vi "IV_Reader_SweepScroller.vi"() -> ()   [LabVIEW 2016]
panel:
  in  "Sweep parameters":T1={"Vbg"=15.0, "Vbg step"=0.0, "Vsg"=-0.5, "Vsg step"=0.025, "B"=0.0, "B step"=0.0, "Temp"=2.0, "Temp step"=0.0}
  in  "PNG output folder":path=path "C:/Users/ansom/Desktop/Agilent/PNG's From Graphs/B_BG_7to-7"
  in  "Large Sweep Folder":path=path "B:/SketchSET/SA03008H.20180718/77_B+SG_B_-7to0inc1_SG_-0.5to0.5inc0.25_at0.2Hz_-300mVto-100mV_IV_@BG15"
  in  "# Fast Sweep":dbl=41.0
  in  "# Slow Sweep":dbl=8.0
  # "Vbg will be updated autmatically"
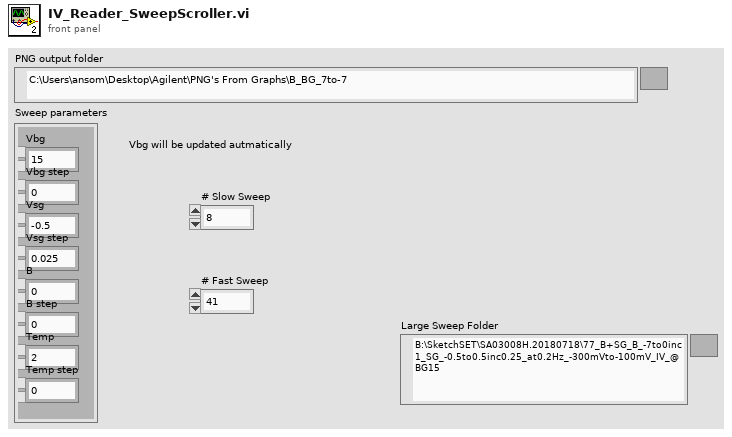
[diagram p1: front panel]
types:
  T1 = cluster{"Vbg":dbl, "Vbg step":dbl, "Vsg":dbl, "Vsg step":dbl, "B":dbl, "B step":dbl, "Temp":dbl, "Temp step":dbl}
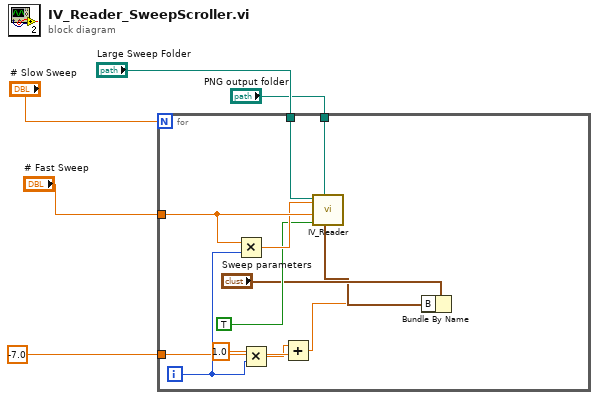
[diagram p0: block diagram]
diagram:
  n1 = for {
    N: "# Slow Sweep" -> [_]
    tunnel: "# Fast Sweep" -> [w17]
    tunnel: "Large Sweep Folder" -> [w15]
    tunnel: "PNG output folder" -> [w13]
    tunnel: -7.0 -> [w8]
    i -> [w9]
    n2 = Multiply(x=w17, y=w9) -> (x*y=w16:dbl)
    n3 = Multiply(x=1.0, y=w9) -> (x*y=w7:dbl)
    n4 = Add(x=w7, y=w8) -> (x+y=w6:dbl)
    n5 = Bundle By Name(cluster="Sweep parameters", "B"=w6) -> (w11:T1)
    n6 = call "IV_Reader.vi"("Sweep parameters"=w11, "Path to PNG Folder"=w13, "Use only a subset of the folder"=TRUE ("Use File Offset"), "Subset Length"=w17, "Subset Index"=w16, "Folder or File"=w15) -> ()  [unwired: 6 in]
  }
